vi "Graph Result.vi"(9 "Reset":bool, 10 "Peak Burst Power":dbl, 11 "Average RMS DEVM %":dbl) -> (2 "appended array":dbl[][](graph))   [LabVIEW 2014, in "niDTS BT.lvlib"]
uses:
  niDTS BT.lvlib
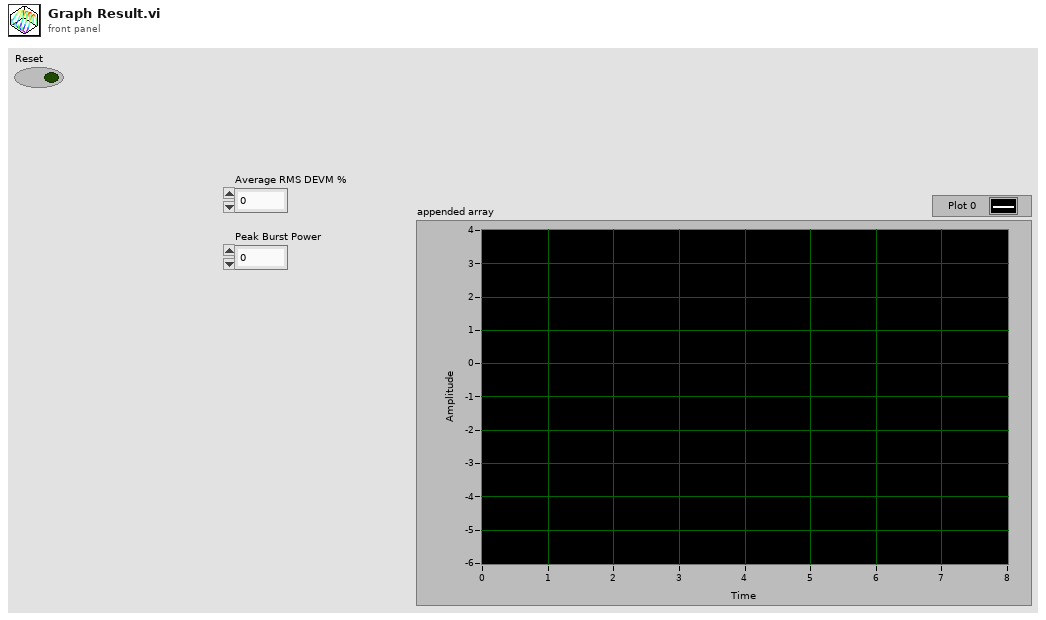
[diagram p1: front panel]
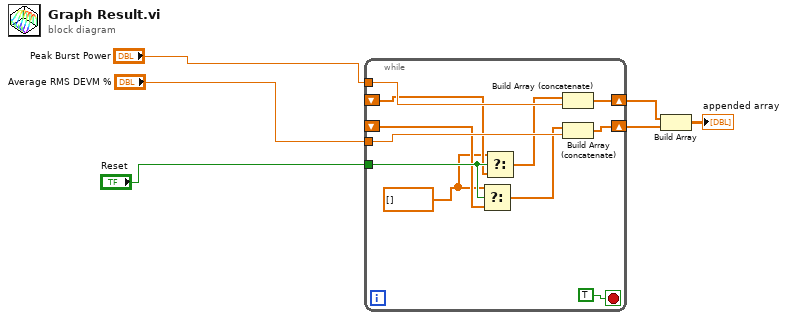
[diagram p0: block diagram]
diagram:
  n1 = while {
    shift-right: [w16] -> w6
    shift-left: _ -> [w11]
    shift-right: [w13] -> w5
    shift-left: _ -> [w9]
    tunnel: "Average RMS DEVM %" -> [w14]
    tunnel: "Peak Burst Power" -> [w15]
    tunnel: "Reset" -> [w12]
    stop <- TRUE stop-if-true
    w7 = dbl[] [] ("t")
    n2 = Select(t=w7, s=w12, f=w9) -> (s? t:f=w8:dbl[])
    n3 = Select(t=w7, s=w12, f=w11) -> (s? t:f=w10:dbl[])
    n4 = Build Array (concatenate)(w10, w15) -> (w16:dbl[])
    n5 = Build Array (concatenate)(w8, w14) -> (w13:dbl[])
  }
  n6 = Build Array(w6, w5) -> (→"appended array":dbl[][])
